vi "YearMonth2Timestamp.vi"(10 "Month":i32, 11 "Year":i32) -> (3 "Time Stamp":timestamp)   [LabVIEW 2017, in "UI_TimeSelector.xctl"]
uses:
  UI_TimeSelector/UI_TimeSelector.xctl
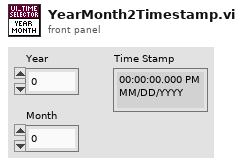
[diagram p1: front panel]
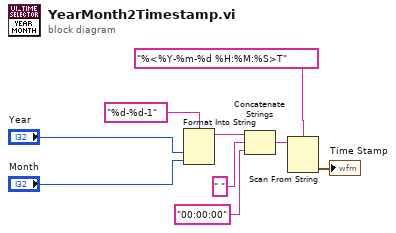
[diagram p0: block diagram]
diagram:
  n1 = Format Into String(format string="%d-%d-1", "Year", "Month") -> (resulting string=w1:string)  [unwired: 2 in, 1 out]
  n2 = Concatenate Strings(w1, " " ("string"), "00:00:00" ("string")) -> (w7:string)
  n3 = Scan From String(format string="%<%Y-%m-%d %H:%M:%S>T", input string=w7) -> (output 1=→"Time Stamp":timestamp)  [unwired: 3 in, 3 out]
